vi "From CSV File.vi"(8 "error in (no error)":errorcluster, 9 "Path":path, 10 "engine in":refnum<class "engine configuration.lvclass">, 11 "tag bus configurable plugin editor node in":refnum<class "tag bus configurable plugin editor node.lvclass">) -> (0 "error out":errorcluster, 1 "Update":bool, 2 "engine out":refnum<class "engine configuration.lvclass">, 3 "tag bus configurable plugin editor node out":refnum<class "tag bus configurable plugin editor node.lvclass">)   [LabVIEW 2014, in "tag bus configurable plugin editor node.lvclass"]
uses:
  tag bus configurable plugin editor node.lvclass
  <vilib>/NI/Module Execution Interface/Engine Configuration/engine configuration.lvclass
  module/configuration/tag bus configurable plugin module configuration.lvclass
  <vilib>/NI/Configuration Framework/serializable configuration/NISE_CEF_serializable configuration.lvclass/NISE_CEF_serializable configuration.ctl
  module/configuration/tag bus configurable plugin module configuration.lvclass/tag bus configurable plugin module configuration.ctl
  <vilib>/NI/Tag Bus/tag/tag descriptor.lvclass/tag descriptor.ctl
  <vilib>/Utility/LVClass/Get LV Class Name.vi
  <vilib>/NI/Configuration Framework/error generator/NISE_error generator.vi
  <vilib>/NI/Tag Bus Module Framework/channel/TBM channel.lvclass
  <vilib>/NI/Configuration Framework/serializable configuration/NISE_CEF_serializable configuration.lvclass
  <vilib>/NI/Tag Bus/tag/tag descriptor.lvclass
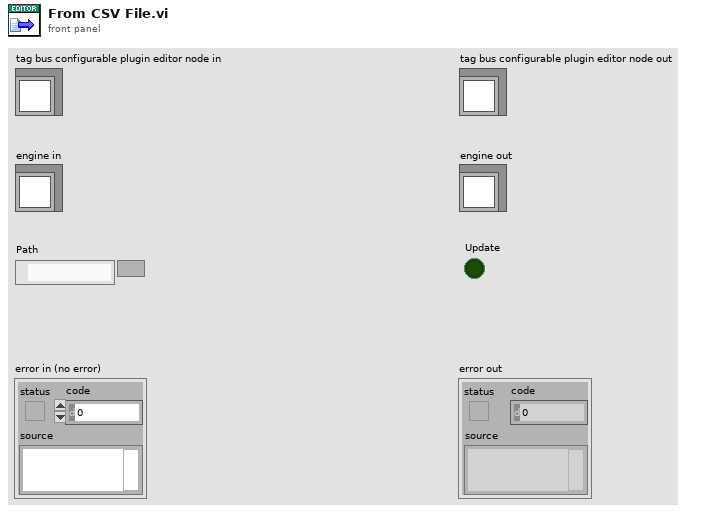
[diagram p1: front panel]
types:
  T1 = typedef "tag bus configurable plugin module configuration.lvclass/Line.ctl" = cluster{"channel":refnum<class "TBM channel.lvclass">}
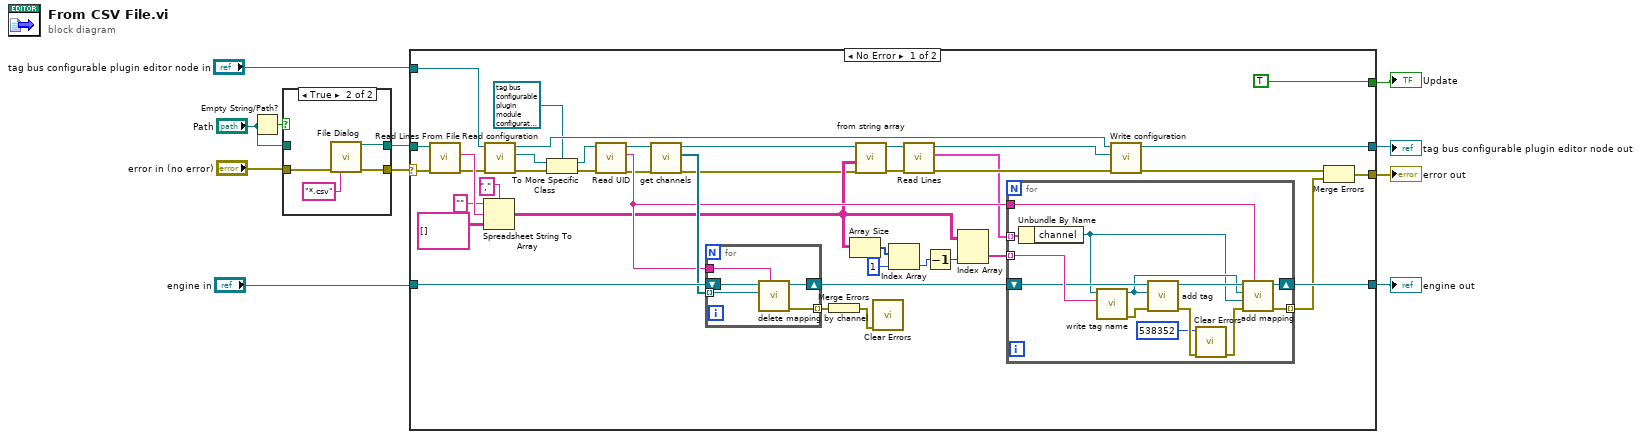
[diagram p0: block diagram]
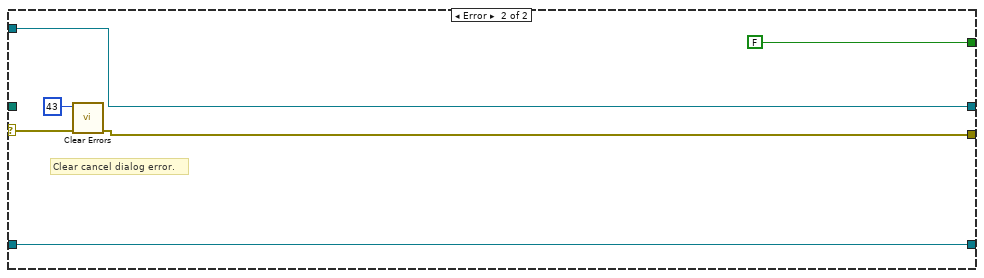
[diagram p2: hidden frame]
diagram:
  n1 = Empty String/Path?(string/path="Path") -> (empty?=w11:bool)
  n2 = case shown="True" w11 {
    tunnel: "error in (no error)" -> [w12 w16]
    tunnel: [w12 w15] -> w7
    tunnel: [w13 w14] -> w8
    tunnel: "Path" -> [w13 _]
    frame False {
    }
    frame True {
      n3 = call "File Dialog"("error in"=w16, "pattern (all files)"="*.csv") -> ("selected path"=w14:path, "error out"=w15:errorcluster)  [unwired: 10 in, 2 out]
    }
  }
  n4 = case shown="No Error" w7 {
    selector: w7 -> [w51 w79]
    tunnel: [w39 w78] -> w1
    tunnel: [w27 w81] -> w3
    tunnel: "tag bus configurable plugin editor node in" -> [w32 w81]
    tunnel: w8 -> [w56 _]
    tunnel: [TRUE ("Update") FALSE ("Update")] -> w4
    tunnel: "engine in" -> [w48 w76]
    tunnel: [w41 w76] -> w2
    frame No Error {
      n5 = call <vilib>:"Read Lines From File.vi"("file path (dialog if empty)"=w56, "error in (not an error)"=w51) -> ("line string"=w54:string, "error out"=w31:errorcluster)  [unwired: 5 in, 1 out]
      n6 = Spreadsheet String To Array(delimiter (Tab)=",", format string="", spreadsheet string=w54, array type (2D Dbl)=string[][] [] ("type (empty)")) -> (array=w37:string[][])
      n7 = call-dynamic "Read configuration.vi"("error in"=w31, "tag bus configurable plugin editor node in"=w32) -> ("error out"=w29:errorcluster, "configuration"=w30:refnum<class "NISE_CEF_serializable configuration.lvclass">, "tag bus configurable plugin editor node out"=w28:refnum<class "tag bus configurable plugin editor node.lvclass">)  [unwired: 7 in]
      n8 = To More Specific Class(target class=refnum<class "tag bus configurable plugin module configuration.lvclass"> refnum ("tag bus configurable plugin module configuration"), reference=w30, error in=w29) -> (specific class reference=w50:refnum<class "tag bus configurable plugin module configuration.lvclass">, error out=w44:errorcluster)
      n9 = call <vilib>:"Read UID.vi"("error in"=w44, "configuration in"=w50) -> ("error out"=w24:errorcluster, "instance id"=w40:string, "configuration out"=w49:refnum<class "tag bus configurable plugin module configuration.lvclass">)  [unwired: 7 in]
      n10 = call-dynamic "get channels.vi"("module configuration in"=w49) -> ("channels"=w47:refnum<class "TBM channel.lvclass">[], "module configuration out"=w45:refnum<class "tag bus configurable plugin module configuration.lvclass">)  [unwired: 9 in]
      n11 = for {
        tunnel: w40 -> [w74]
        tunnel: w47 -> [w73] mode=indexing
        tunnel: [w72] -> w46 mode=indexing
        shift-right: [w71] -> w42
        shift-left: w48 -> [w75]
        n12 = call <vilib>:"delete mapping by channel.vi"("owner ID"=w74, "channel"=w73, "engine configuration in"=w75) -> ("error out"=w72:errorcluster, "engine configuration out"=w71:refnum<class "engine configuration.lvclass">)  [unwired: 7 in]
      }
      n13 = Merge Errors(w46) -> (w25:errorcluster)
      n14 = Array Size(array=w37) -> (size(s)=w36:i32[])
      n15 = call-dynamic "from string array.vi"("error in (no error)"=w24, "String Array"=w37, "module configuration in"=w45) -> ("error out"=w22:errorcluster, "module configuration out"=w18:refnum<class "tag bus configurable plugin module configuration.lvclass">)  [unwired: 7 in]
      n16 = call <vilib>:"Clear Errors.vi"("error in (no error)"=w25) -> ()  [unwired: 5 in, 2 out]
      n17 = Index Array(array=w36, index=1) -> (element=w34:i32)
      n18 = call "Read Lines.vi"("error in (no error)"=w22, "tag bus configurable plugin module configuration in"=w18) -> ("error out"=w21:errorcluster, "Lines"=w20:T1[], "tag bus configurable plugin module configuration out"=w19:refnum<class "tag bus configurable plugin module configuration.lvclass">)  [unwired: 7 in]
      n19 = Decrement(x=w34) -> (x-1=w33:i32)
      n20 = Index Array(array=w37, index (col)=w33) -> (element=w43:string[])  [unwired: 1 in]
      n21 = for {
        tunnel: w20 -> [w70] mode=indexing
        tunnel: w43 -> [w69] mode=indexing
        shift-right: [w68] -> w41
        shift-left: w42 -> [w65]
        tunnel: w40 -> [w67]
        tunnel: [w66] -> w38 mode=indexing
        n22 = Unbundle By Name(w70) -> ("channel"=w62:refnum<class "TBM channel.lvclass">)
        n23 = call <vilib>:"write tag name.vi"("name"=w69, "system tag in"=w62) -> ("error out"=w61:errorcluster, "system tag out"=w63:refnum<class "TBM channel.lvclass">)  [unwired: 8 in]
        n24 = call-dynamic "add tag.vi"("error in"=w61, "tag descriptor"=w63, "engine configuration in"=w65) -> ("error out"=w60:errorcluster, "engine configuration out"=w64:refnum<class "engine configuration.lvclass">)  [unwired: 7 in]
        n25 = call <vilib>:"Clear Errors.vi"("error in (no error)"=w60, "specific error code to clear (0: all)"=538352) -> ("error out"=w59:errorcluster)  [unwired: 4 in, 1 out]
        n26 = call-dynamic "add mapping.vi"("owner ID"=w67, "error in"=w59, "channel"=w62, "tag descriptor"=w63, "engine configuration"=w64) -> ("error out"=w66:errorcluster, "engine configuration out"=w68:refnum<class "engine configuration.lvclass">)  [unwired: 5 in]
      }
      n27 = call-dynamic "Write configuration.vi"("error in"=w21, "configuration"=w19, "tag bus configurable plugin editor node in"=w28) -> ("error out"=w26:errorcluster, "tag bus configurable plugin editor node out"=w27:refnum<class "tag bus configurable plugin editor node.lvclass">)  [unwired: 7 in]
      n28 = Merge Errors(w26, w38) -> (w39:errorcluster)
    }
    frame Error {
      # "Clear cancel dialog error."
      n29 = call <vilib>:"Clear Errors.vi"("error in (no error)"=w79, "specific error code to clear (0: all)"=43) -> ("error out"=w78:errorcluster)  [unwired: 4 in, 1 out]
    }
  }
  "error out" <- w1
  "tag bus configurable plugin editor node out" <- w3
  "Update" <- w4
  "engine out" <- w2
